vi "ReadLookup.vi"(8 "IntenOff":u32, 11 "RefIn":refnum<file>) -> (0 "Lookup":u32[](array[numeric]), 3 "RefOut":refnum<file>)   [LabVIEW 2012]
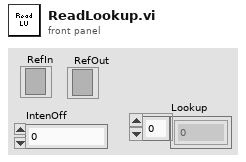
[diagram p1: front panel]
types:
  T1 = enum16{"big-endian, network order", "native, host order", "little-endian"}
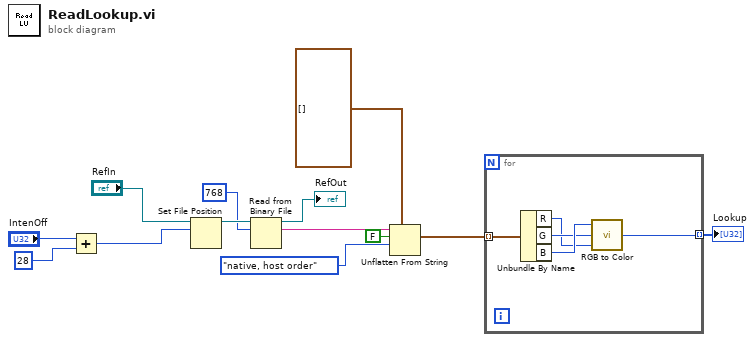
[diagram p0: block diagram]
diagram:
  n1 = Add(x="IntenOff", y=u32 28) -> (x+y=w10:u32)
  n2 = Set File Position(offset (in bytes) (0)=w10, refnum="RefIn") -> (refnum out=w9:refnum<file>)  [unwired: 2 in, 1 out]
  n3 = Read from Binary File(10:768 ("count (1)"), 11:w9) -> (2:w6:string, 3:→"RefOut":refnum<file>)  [unwired: 4 in, 2 out]
  n4 = Unflatten From String(type=cluster{"R":u8, "G":u8, "B":u8}[] [], binary string=w6, data includes array or string size? (T)=FALSE, byte order (0:big-endian, network order)=T1."native, host order") -> (value=w2:cluster{"R":u8, "G":u8, "B":u8}[])  [unwired: 1 in, 2 out]
  n5 = for {
    tunnel: w2 -> [w18] mode=indexing
    tunnel: [w14] -> w1 mode=indexing
    n6 = Unbundle By Name(w18) -> ("R"=w15:u8, "G"=w16:u8, "B"=w17:u8)
    n7 = call <vilib>:"RGB to Color.vi"("B"=w15, "G"=w16, "R"=w17) -> ("Color"=w14:u32)
  }
  "Lookup" <- w1
